vi "AddChild.vi"(8 "error in (no error)":errorcluster, 10 "Object":refnum<class "Pgui_Obj.lvclass">, 11 "reference in":refnum<class "Pgui_Obj.lvclass">) -> (0 "error out":errorcluster, 3 "reference out":refnum<class "Pgui_Obj.lvclass">)   [LabVIEW 2019, in "Pgui_Obj.lvclass"]
doc: "Adds Child object root must be passed in to keep track of parent."
uses:
  Pgui_Obj.lvclass
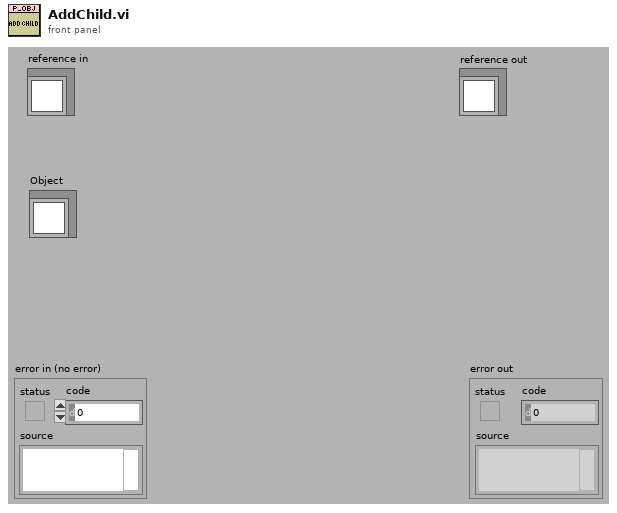
[diagram p1: front panel]
types:
  T1 = typedef "Pgui_Obj.lvclass/ObjectAttributes.ctl" = cluster{"Children":refnum<class "Pgui_Obj.lvclass">[], "Draw Instr":picture, "Params":cluster{"left":i16, "top":i16, "right":i16, "bottom":i16}, "Parent_Pgui_Obj":refnum<class "Pgui_Obj.lvclass">, "MouseOver":bool}
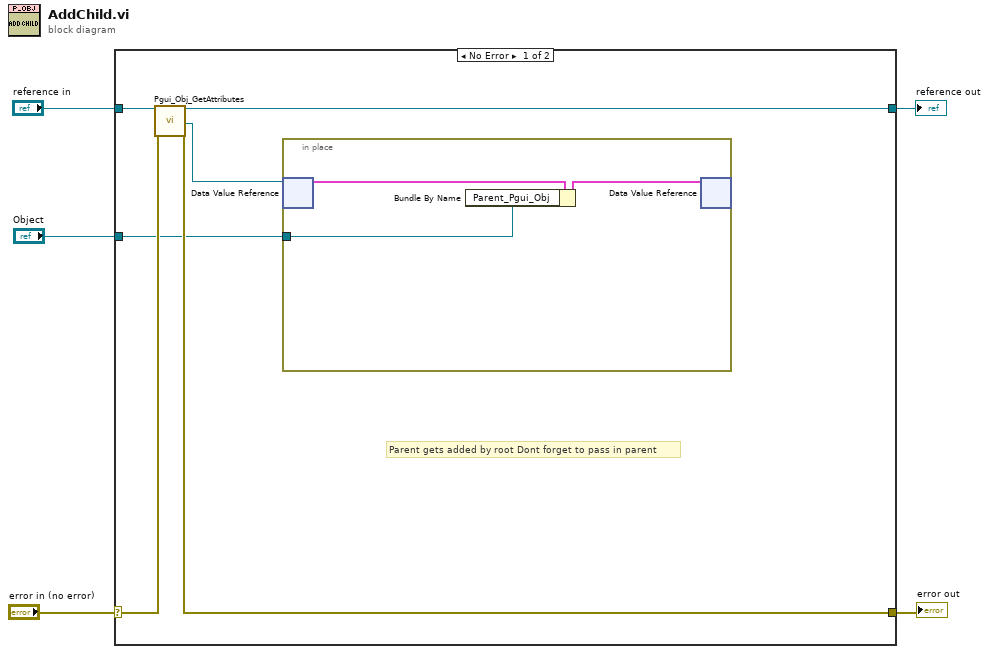
[diagram p0: block diagram]
diagram:
  n1 = case shown="No Error" "error in (no error)" {
    selector: "error in (no error)" -> [w11 w16]
    tunnel: [w10 w16] -> w4
    tunnel: [w8 w15] -> w2
    tunnel: "reference in" -> [w9 w15]
    tunnel: "Object" -> [w6 _]
    frame No Error {
      # "Parent gets added by root Dont forget to pass in parent"
      n2 = call "Pgui_Obj_GetAttributes.vi"("reference in"=w9, "error in (no error)"=w11) -> ("reference out"=w8:refnum<class "Pgui_Obj.lvclass">, "DataRef"=w7:refnum<data-value>, "error out"=w10:errorcluster)  [unwired: 14 in, 1 out]
      n3 = in-place {
        in-place-border: w6 -> [w12]
        n4 = in-place-dvr #1(w7) -> (w14:T1)  [unwired: 1 out]
        n5 = Bundle By Name(cluster=w14, "Parent_Pgui_Obj"=w12) -> (w13:T1)
        n6 = in-place-dvr #1(w13) -> ()  [unwired: 2 out]
      }
    }
    frame Error {
    }
  }
  "error out" <- w4
  "reference out" <- w2
